vi "AddNewFlexUIActorClassToLibrary.vi"(8 "error in (no error)":errorcluster, 11 "FlexUIActorMaker in":refnum<class "FlexUIActorMaker.lvclass">) -> (0 "error out":errorcluster, 3 "FlexUIActorMaker out":refnum<class "FlexUIActorMaker.lvclass">)   [LabVIEW 2016, in "FlexUIActorMaker.lvlib" / "FlexUIActorMaker.lvclass"]
uses:
  FlexUIActorMaker.lvclass
  FlexUIActorMaker.lvclass/FlexUIActorMaker.ctl
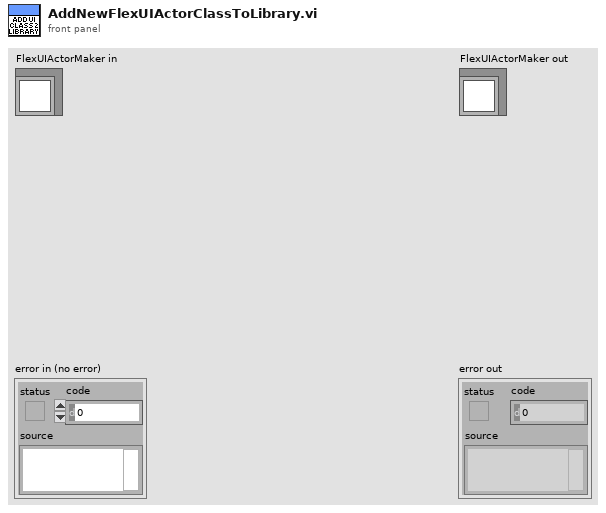
[diagram p1: front panel]
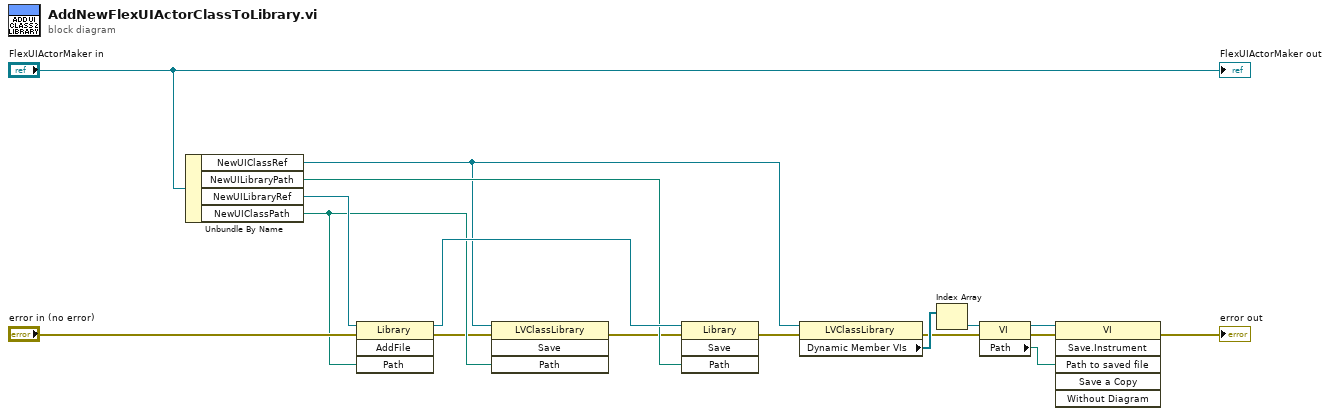
[diagram p0: block diagram]
diagram:
  n1 = Unbundle By Name("FlexUIActorMaker in") -> ("NewUIClassRef"=w7:refnum<vi>, "NewUILibraryPath"=w13:path, "NewUILibraryRef"=w15:refnum<vi>, "NewUIClassPath"=w12:path)
  n2 = invoke class="Library" method="AddFile"(reference=w15, error in="error in (no error)", "Path"=w12) -> (reference out=w14:refnum<vi>, error out=w10:errorcluster)  [unwired: 1 in, 2 out]
  n3 = invoke class="LVClassLibrary" method="Save"(reference=w7, error in=w10, "Path"=w12) -> (error out=w11:errorcluster)  [unwired: 1 in, 3 out]
  n4 = invoke class="Library" method="Save"(reference=w14, error in=w11, "Path"=w13) -> (error out=w9:errorcluster)  [unwired: 1 in, 3 out]
  n5 = property class="LVClassLibrary"(reference=w7, error in=w9) -> (error out=w3:errorcluster, "Dynamic Member VIs"=w8:refnum<vi>[])  [unwired: 1 out]
  n6 = Index Array(array=w8) -> (element=w6:refnum<vi>)  [unwired: 1 in]
  n7 = property class="VI"(reference=w6, error in=w3) -> (reference out=w5:refnum<vi>, error out=w2:errorcluster, "Path"=w4:path)
  n8 = invoke class="VI" method="Save.Instrument"(reference=w5, error in=w2, "Path to saved file"=w4) -> (error out=→"error out":errorcluster)  [unwired: 3 in, 5 out]
  "FlexUIActorMaker out" <- "FlexUIActorMaker in"
